vi "GetFailureRateFromDigitalCtrl.vi"(10 "defective digital ref":refnum<vi>, 11 "checking count digital ref":refnum<vi>) -> (3 "result":string)   [LabVIEW 2018, in "Library-Ctrl.lvlib"]
uses:
  Library-Ctrl.lvlib
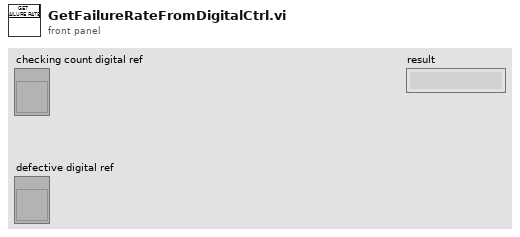
[diagram p1: front panel]
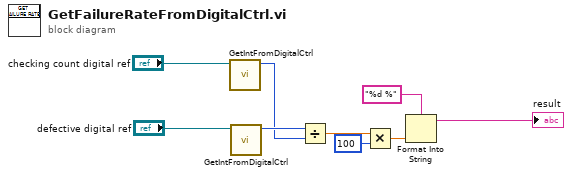
[diagram p0: block diagram]
diagram:
  n1 = call "GetIntFromDigitalCtrl.vi"("int value ref"="checking count digital ref") -> ("result"=w6:i32)  [unwired: 10 in]
  n2 = call "GetIntFromDigitalCtrl.vi"("int value ref"="defective digital ref") -> ("result"=w7:i32)  [unwired: 10 in]
  n3 = Divide(x=w7, y=w6) -> (x/y=w5:dbl)
  n4 = Multiply(x=w5, y=100) -> (x*y=w2:dbl)
  n5 = Format Into String(format string="%d %" ("포맷 문자열"), w2) -> (resulting string=→"result":string)  [unwired: 2 in, 1 out]
